vi "Untitled 4 (SubVI).vi"(11 "Output Array":string[][](array[string])) -> (0 "mean":dbl format="%0.2f", 1 "output 3":u16, 2 "output 2":dbl format="%.2f", 3 "rms value":dbl format="%0.2f", 4 "(hi.lo)":u64, 5 "odeslana predkosc":u16, 6 "war reg":u32)   [LabVIEW 2015]
uses:
  <vilib>/ptbypt/NI_PtbyPt.lvlib
panel:
  out "element 2":string
  out "x << y 2":u32
  out "(hi.lo) 5":u16
  out "(hi.lo) 4":u16 format="%b"
  out "unsigned 8bit integer 2":u8 format="%b"
  out "unsigned 8bit integer":u8 format="%b"
  out "(hi.lo) 3":u16 format="%b"
  out "(hi.lo) 2":u16
  out "x << y":u32
  out "element":string
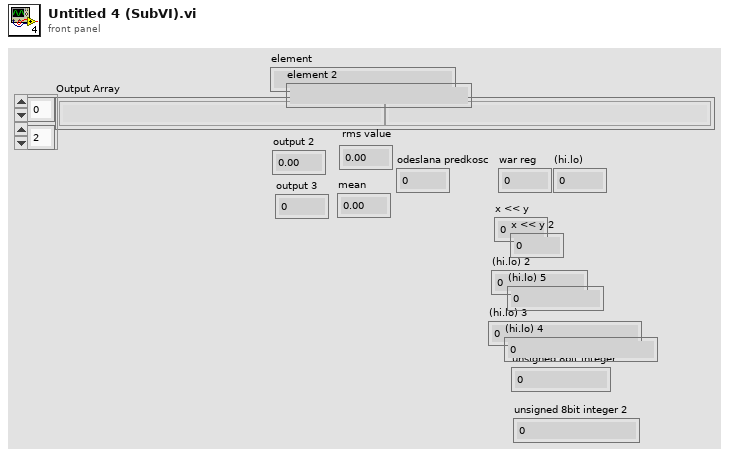
[diagram p1: front panel]
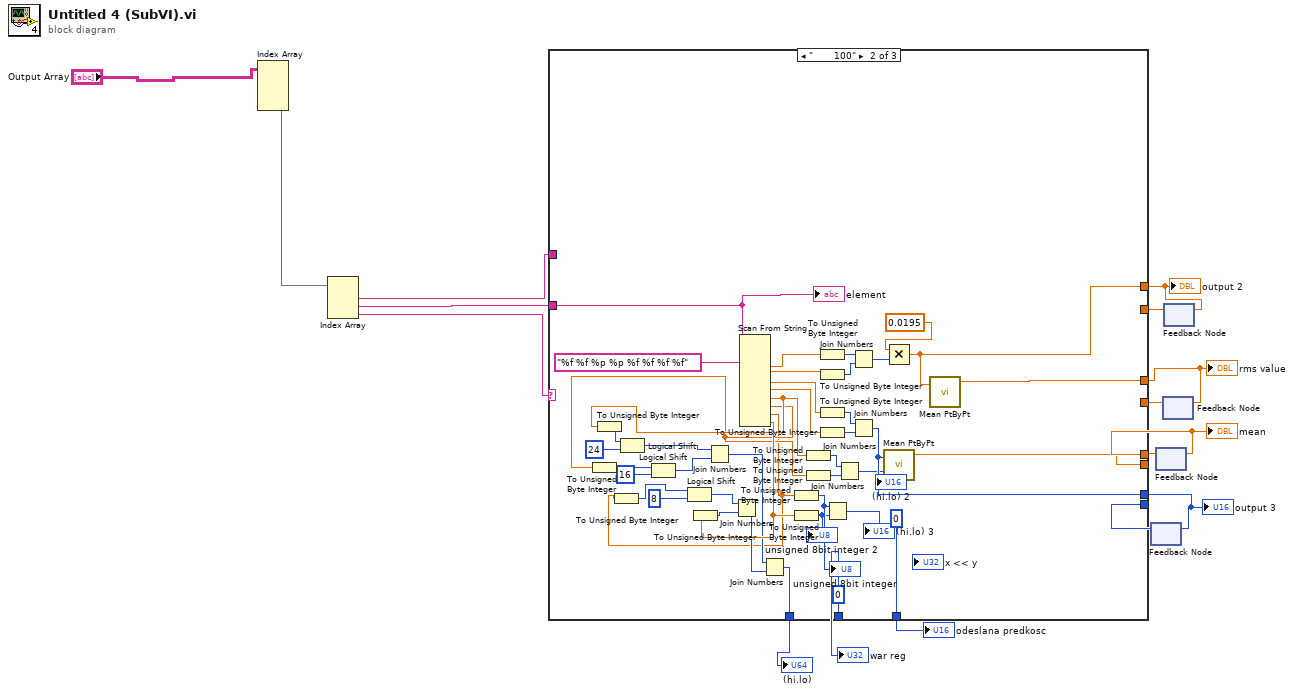
[diagram p0: block diagram]
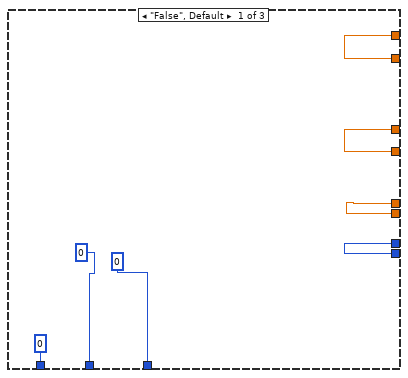
[diagram p2: hidden frame]
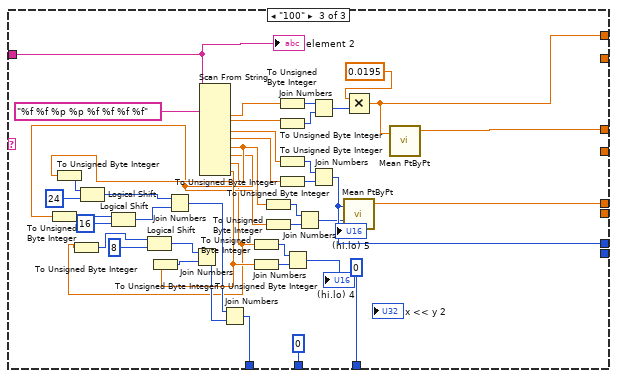
[diagram p3: hidden frame]
diagram:
  n1 = Index Array(array="Output Array") -> (element #2=w15:string[])  [unwired: 4 in, 1 out]
  n2 = Index Array(array=w15) -> (element #1=w1:string, element #2=w14:string, element #3=w13:string)  [unwired: 3 in]
  n3 = feedback #1() -> (w5:u16)  [unwired: 1 in]
  n4 = feedback #2() -> (w10:dbl)  [unwired: 1 in]
  n5 = feedback #3() -> (w9:dbl)  [unwired: 1 in]
  n6 = feedback #4() -> (w6:dbl)  [unwired: 1 in]
  n7 = case shown="\"       100\"" w13 {
    tunnel: w14 -> [_ w54 w95]
    tunnel: [w22 w52 w93] -> w12
    tunnel: [w23 w51 w92] -> w11
    tunnel: w10 -> [w23 _ _]
    tunnel: w9 -> [w22 _ _]
    tunnel: [w21 w50 w91] -> w7
    tunnel: [w20 w49 w90] -> w8
    tunnel: w6 -> [w21 _ _]
    tunnel: w5 -> [w20 _ _]
    tunnel: [u16 0 u16 0 u16 0] -> w4
    tunnel: [u16 0 u16 0 u16 0] -> w3
    tunnel: [u64 0 w27 w68] -> w2
    tunnel: w1 -> [_ _ _]
    frame "False", Default {
    }
    frame "       100" {
      n8 = Scan From String(format string="%f %f %p %p %f %f %f %f", input string=w54) -> (output 1=w62:dbl, output 2=w61:dbl, output 3=w60:dbl, output 4=w57:dbl, output 5=w34:dbl, output 6=w31:dbl, output 7=w28:dbl, output 8=w36:dbl)  [unwired: 10 in, 3 out]
      n9 = To Unsigned Byte Integer(number=w31) -> (unsigned 8bit integer=w30:u8)
      n10 = To Unsigned Byte Integer(number=w34) -> (unsigned 8bit integer=w35:u8)
      n11 = To Unsigned Byte Integer(number=w28) -> (unsigned 8bit integer=w29:u8)
      n12 = Logical Shift(y=w35, x=u32 24) -> (x << y=w40:u32)
      n13 = Logical Shift(y=w30, x=u32 16) -> (x << y=w39:u32)
      n14 = Logical Shift(y=w29, x=u32 8) -> (x << y=w38:u32)
      n15 = To Unsigned Byte Integer(number=w36) -> (unsigned 8bit integer=w37:u8)
      n16 = Join Numbers(hi=w40, lo=w39) -> ((hi.lo)=w33:u64)
      n17 = Join Numbers(hi=w38, lo=w37) -> ((hi.lo)=w32:u64)
      n18 = Join Numbers(hi=w33, lo=w32) -> ((hi.lo)=w27:u64)
      n19 = To Unsigned Byte Integer(number=w28) -> (unsigned 8bit integer=w46:u8)
      "unsigned 8bit integer" <- w46
      n20 = To Unsigned Byte Integer(number=w36) -> (unsigned 8bit integer=w45:u8)
      "unsigned 8bit integer 2" <- w45
      n21 = To Unsigned Byte Integer(number=w34) -> (unsigned 8bit integer=w47:u8)
      n22 = To Unsigned Byte Integer(number=w31) -> (unsigned 8bit integer=w48:u8)
      n23 = To Unsigned Byte Integer(number=w62) -> (unsigned 8bit integer=w59:u8)
      n24 = To Unsigned Byte Integer(number=w61) -> (unsigned 8bit integer=w58:u8)
      n25 = To Unsigned Byte Integer(number=w60) -> (unsigned 8bit integer=w56:u8)
      n26 = To Unsigned Byte Integer(number=w57) -> (unsigned 8bit integer=w55:u8)
      n27 = Join Numbers(hi=w46, lo=w45) -> ((hi.lo)=→"(hi.lo) 3":u16)
      n28 = Join Numbers(hi=w47, lo=w48) -> ((hi.lo)=→"(hi.lo) 2":u16)
      n29 = Join Numbers(hi=w59, lo=w58) -> ((hi.lo)=w53:u16)
      n30 = Join Numbers(hi=w56, lo=w55) -> ((hi.lo)=w49:u16)
      n31 = Multiply(x=0.0195, y=w53) -> (x*y=w50:dbl)
      n32 = call <vilib>:"Mean PtByPt.vi"("x"=w49) -> ("mean"=w51:dbl)  [unwired: 3 in, 1 out]
      n33 = call <vilib>:"Mean PtByPt.vi"("x"=w50) -> ("mean"=w52:dbl)  [unwired: 3 in, 1 out]
      "element" <- w54
    }
    frame "100" {
      n34 = Scan From String(format string="%f %f %p %p %f %f %f %f", input string=w95) -> (output 1=w103:dbl, output 2=w102:dbl, output 3=w101:dbl, output 4=w98:dbl, output 5=w75:dbl, output 6=w72:dbl, output 7=w69:dbl, output 8=w77:dbl)  [unwired: 10 in, 3 out]
      n35 = To Unsigned Byte Integer(number=w72) -> (unsigned 8bit integer=w71:u8)
      n36 = To Unsigned Byte Integer(number=w75) -> (unsigned 8bit integer=w76:u8)
      n37 = To Unsigned Byte Integer(number=w69) -> (unsigned 8bit integer=w70:u8)
      n38 = Logical Shift(y=w76, x=u32 24) -> (x << y=w81:u32)
      n39 = Logical Shift(y=w71, x=u32 16) -> (x << y=w80:u32)
      n40 = Logical Shift(y=w70, x=u32 8) -> (x << y=w79:u32)
      n41 = To Unsigned Byte Integer(number=w77) -> (unsigned 8bit integer=w78:u8)
      n42 = Join Numbers(hi=w81, lo=w80) -> ((hi.lo)=w74:u64)
      n43 = Join Numbers(hi=w79, lo=w78) -> ((hi.lo)=w73:u64)
      n44 = Join Numbers(hi=w74, lo=w73) -> ((hi.lo)=w68:u64)
      n45 = To Unsigned Byte Integer(number=w69) -> (unsigned 8bit integer=w87:u8)
      n46 = To Unsigned Byte Integer(number=w77) -> (unsigned 8bit integer=w86:u8)
      n47 = To Unsigned Byte Integer(number=w75) -> (unsigned 8bit integer=w88:u8)
      n48 = To Unsigned Byte Integer(number=w72) -> (unsigned 8bit integer=w89:u8)
      n49 = To Unsigned Byte Integer(number=w103) -> (unsigned 8bit integer=w100:u8)
      n50 = To Unsigned Byte Integer(number=w102) -> (unsigned 8bit integer=w99:u8)
      n51 = To Unsigned Byte Integer(number=w101) -> (unsigned 8bit integer=w97:u8)
      n52 = To Unsigned Byte Integer(number=w98) -> (unsigned 8bit integer=w96:u8)
      n53 = Join Numbers(hi=w87, lo=w86) -> ((hi.lo)=→"(hi.lo) 4":u16)
      n54 = Join Numbers(hi=w88, lo=w89) -> ((hi.lo)=→"(hi.lo) 5":u16)
      n55 = Join Numbers(hi=w100, lo=w99) -> ((hi.lo)=w94:u16)
      n56 = Join Numbers(hi=w97, lo=w96) -> ((hi.lo)=w90:u16)
      n57 = Multiply(x=0.0195, y=w94) -> (x*y=w91:dbl)
      n58 = call <vilib>:"Mean PtByPt.vi"("x"=w90) -> ("mean"=w92:dbl)  [unwired: 3 in, 1 out]
      n59 = call <vilib>:"Mean PtByPt.vi"("x"=w91) -> ("mean"=w93:dbl)  [unwired: 3 in, 1 out]
      "element 2" <- w95
    }
  }
  "rms value" <- w12
  "mean" <- w11
  "output 2" <- w7
  "output 3" <- w8
  "odeslana predkosc" <- w4
  "war reg" <- w3
  "(hi.lo)" <- w2
  n60 = feedback-in #1(w8) -> ()
  n61 = feedback-in #2(w11) -> ()
  n62 = feedback-in #3(w12) -> ()
  n63 = feedback-in #4(w7) -> ()
